vi "Close Spartan Database.vi"(6 "Force Close? (f)":bool, 8 "error in (no error)":errorcluster, 11 "Connection Refnum":T1) -> (0 "error out":errorcluster)   [LabVIEW 2011]
uses:
  Summitek/Win32/ODBC/SQL Controls/Connection Refnum.ctl
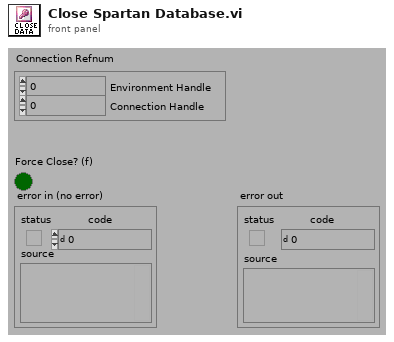
[diagram p1: front panel]
types:
  T1 = typedef "Connection Refnum.ctl" = cluster{"Environment Handle":i32, "Connection Handle":i32}
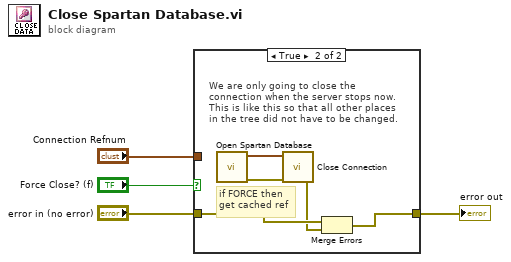
[diagram p0: block diagram]
diagram:
  n1 = case shown="True" "Force Close? (f)" {
    tunnel: "error in (no error)" -> [w5 w10]
    tunnel: [w5 w8] -> w3
    tunnel: "Connection Refnum" -> [_ _]
    frame False {
    }
    frame True {
      # "if FORCE then\nget cached ref"
      # "We are only going to close the\nconnection when the server stops now.\nThis is like this so that all other places\nin the tree did not have to be changed."
      n2 = call "Open Spartan Database.vi"() -> ("error out"=w6:errorcluster, "Connection Refnum"=w7:T1)  [unwired: 10 in]
      n3 = call "Close Connection.vi"("error in (no error)"=w6, "Connection Refnum"=w7) -> ("error out"=w9:errorcluster)  [unwired: 5 out]
      n4 = Merge Errors(w10, w9) -> (w8:errorcluster)
    }
  }
  "error out" <- w3
